vi "Archive.vi"   [LabVIEW 2016]
uses:
  <vilib>/lvdsc/NI_DSC.lvlib
panel:
  # "This VI archive the [Default_Database] on [HousesOfTheHoly] \nto [F_Citadel_Database_Backup] on [CustardPie], every half an\nhour.\n\nThe orignal database will not be deleted by this VI after \nthe copying process."
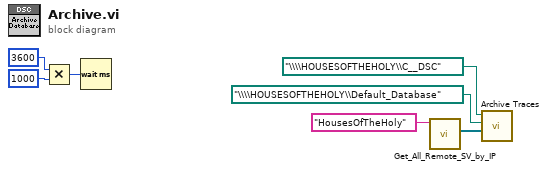
[diagram p0: block diagram]
diagram:
  n1 = Multiply(x=u32 3600, y=u32 1000 ("milliseconds to wait")) -> (x*y=w2:u32)
  n2 = Wait (ms)(milliseconds to wait=w2) -> ()  [unwired: 1 out]
  n3 = call "Get_All_Remote_SV_by_IP.vi"("IP Address"="HousesOfTheHoly") -> ("Shared Variable List"=w6:refnum<k21>[])  [unwired: 8 in, 2 out]
  n4 = call <vilib>:"Archive Traces.vi"("trace names"=w6, "destination database URL"=path "\\\\HOUSESOFTHEHOLY\\Default_Database", "source database URL"=path "\\\\HOUSESOFTHEHOLY\\C__DSC") -> ()  [unwired: 6 in, 3 out]
